vi "Enqueue all axes.vi"(7 "Message":string="Stop", 8 "error in (no error)":errorcluster, 10 "Array":refnum<k21>[](array[refnum]), 11 "Queue in":refnum<queue>) -> (0 "error out":errorcluster, 3 "Queue out":refnum<queue>)   [LabVIEW 2013]
uses:
  support/Message Queue/Message Cluster.ctl
  Typedef/Typedef_Motor_Message.ctl
  EMC API/EMC_Typedef_Motor_Parameters.ctl
  support/Message Queue/Message Queue.lvlib
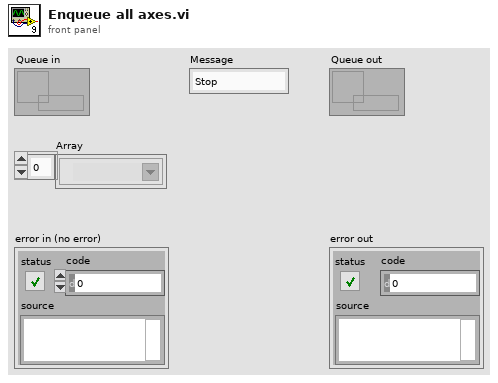
[diagram p1: front panel]
types:
  T1 = typedef "Typedef_Motor_Message.ctl" = cluster{"Axis":refnum<k21>, "Motion Parameters":T2}
  T2 = typedef "EMC_Typedef_Motor_Parameters.ctl" = cluster{"position":dbl, "velocity":dbl, "acceleration":dbl, "deceleration":dbl, "accel. jerk":dbl, "decel. jerk":dbl}
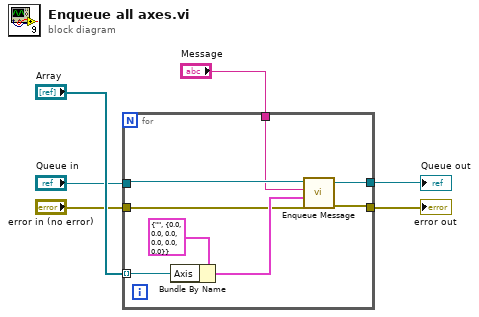
[diagram p0: block diagram]
diagram:
  n1 = for {
    tunnel: "Queue in" -> [w14]
    tunnel: "error in (no error)" -> [w9]
    tunnel: [w8] -> w6
    tunnel: [w13] -> w5
    tunnel: "Array" -> [w10] mode=indexing
    tunnel: "Message" -> [w7]
    n2 = Bundle By Name(cluster=T1 {"Axis"="", "Motion Parameters"={"position"=0.0, "velocity"=0.0, "acceleration"=0.0, "deceleration"=0.0, "accel. jerk"=0.0, "decel. jerk"=0.0}} ("Motor_Message"), "Axis"=w10) -> (w11:T1)
    n3 = call "Enqueue Message.vi"("error in (no error)"=w9, "Message Data"=w11, "Message"=w7, "Message Queue"=w14) -> ("error out"=w8:errorcluster, "dup Message Queue"=w13:refnum<queue>)  [unwired: 6 in]
  }
  "error out" <- w6
  "Queue out" <- w5
